vi "DestroySelfReference.vi"(8 "error in (no error)":errorcluster, 11 "Camera.Simulated":refnum<class "Camera.Simulated.lvclass">) -> (0 "error out":errorcluster, 3 "Camera.Simulated out":refnum<class "Camera.Simulated.lvclass">)   [LabVIEW 2015, in "Camera.Simulated.lvclass"]
doc: "JKI State Machine Objects (SMO) 1.0.0.5\nJKI - JKI\nCopyright (c) 2016, JKI"
uses:
  Camera.Simulated.lvclass
  Camera.Simulated.lvclass/Camera.Simulated.ctl
  Camera/Camera.lvclass
panel:
  # "For instructions on how to use the JKI State Machine Objects, examples and video tutorials, visit:\nhttp://jki.net/state-machine-objects/\n\nJKI State Machine Objects™\nhttp://jki.net/state-machine-objects/\nCopyright (C) 2005-2015, JKI <info@jki.net>\nALL RIGHTS RESERVED"
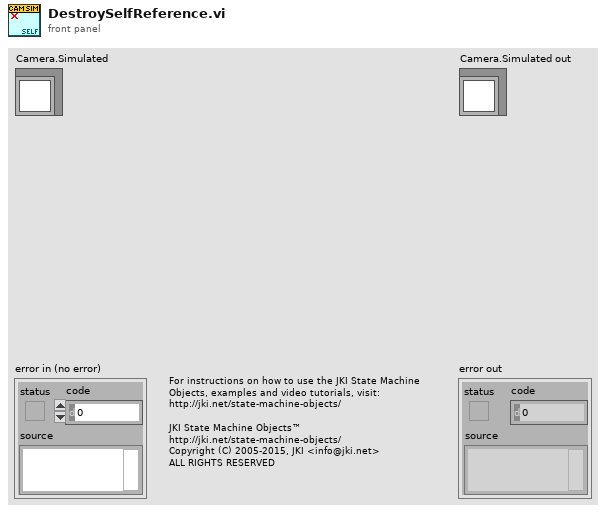
[diagram p1: front panel]
types:
  T1 = typedef "Camera.Simulated.lvclass/PrivateData--Ref.ctl" = refnum<data-value>
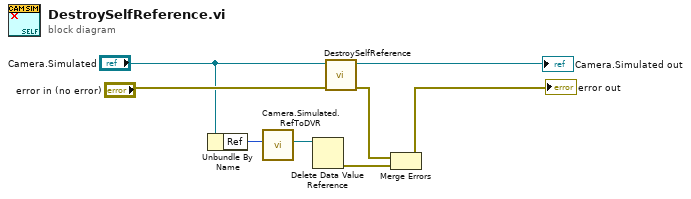
[diagram p0: block diagram]
diagram:
  n1 = Unbundle By Name("Camera.Simulated") -> ("Ref"=w2:u32)
  n2 = call "Camera.Simulated.RefToDVR.vi"("Ref"=w2) -> ("Ref"=w1:T1)  [unwired: 10 in]
  n3 = Delete Data Value Reference(data value reference=w1) -> (error out=w8:errorcluster)  [unwired: 1 in, 1 out]
  n4 = call-parent "DestroySelfReference.vi"("error in (no error)"="error in (no error)", "Camera"="Camera.Simulated") -> ("error out"=w7:errorcluster, "Camera out"=→"Camera.Simulated out":refnum<class "Camera.Simulated.lvclass">)  [unwired: 8 in]
  n5 = Merge Errors(w7, w8) -> (→"error out":errorcluster)
